vi "GetLabels.vi"(0 "Array":T1(array[cluster])) -> (1 "Region Labels":string[](array[string]), 2 "No. of regions":i32, 3 "Strip Labels":string[](array[string]), 4 "No. of Points":i32)   [LabVIEW 2013]
doc: "Utility to read the labels of probe regions and strips."
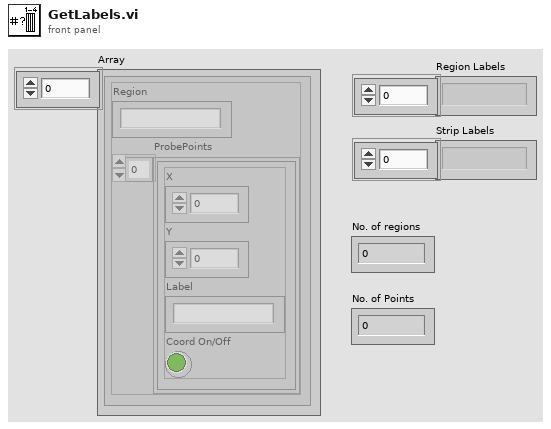
[diagram p1: front panel]
types:
  T1 = cluster{"Region":string, "ProbePoints":cluster{"X":dbl, "Y":dbl, "Label":string, "Coord On/Off":bool}[]}[]
  T2 = cluster{"X":dbl, "Y":dbl, "Label":string, "Coord On/Off":bool}[]
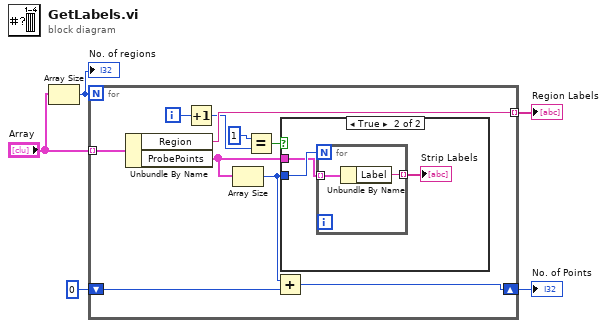
[diagram p0: block diagram]
diagram:
  n1 = Array Size(array="Array") -> (size(s)=w3:i32)
  "No. of regions" <- w3
  n2 = for {
    N: w3 -> [_]
    tunnel: "Array" -> [w15] mode=indexing
    tunnel: [w14] -> w4 mode=indexing
    shift-right: [w10] -> w1
    shift-left: 0 -> [w9]
    i -> [w13]
    n3 = Unbundle By Name(w15) -> ("Region"=w14:string, "ProbePoints"=w7:T2)
    n4 = Increment(x=w13) -> (x+1=w12:i32)
    n5 = Array Size(array=w7) -> (size(s)=w8:i32)
    n6 = Equal?(x=1, y=w12) -> (x = y?=w6:bool)
    n7 = Add(x=w8, y=w9) -> (x+y=w10:i32)
    n8 = case shown="True" w6 {
      tunnel: w8 -> [_ w18]
      tunnel: w7 -> [_ w17]
      frame False {
      }
      frame True {
        n9 = for {
          N: w18 -> [_]
          tunnel: w17 -> [w20] mode=indexing
          tunnel: [w19] -> w16 mode=indexing
          n10 = Unbundle By Name(w20) -> ("Label"=w19:string)
        }
        "Strip Labels" <- w16
      }
    }
  }
  "Region Labels" <- w4
  "No. of Points" <- w1
